vi "GetLibVersionInfo.vi"(8 "error in (no error)":errorcluster, 11 "DLLPath":path) -> (0 "error out":errorcluster, 3 "LibInfo":T1)   [LabVIEW 2022 SP3, in "EClib functions.lvlib"]
doc: "This VI supplies information on the selected DLL:\n- DLL version\n- DLL version string length\n- DLL path"
uses:
  EClib functions.lvlib
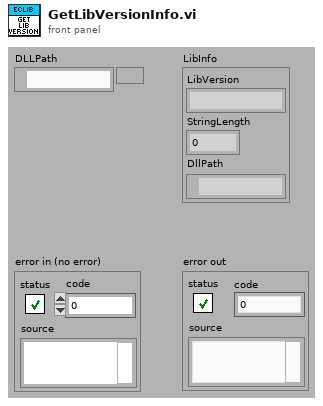
[diagram p1: front panel]
types:
  T1 = cluster{"LibVersion":string, "StringLength":u32, "DllPath":path}
  T2 = cluster{"arg1":string, "arg2":u32, "ECLibDLLPath":path}
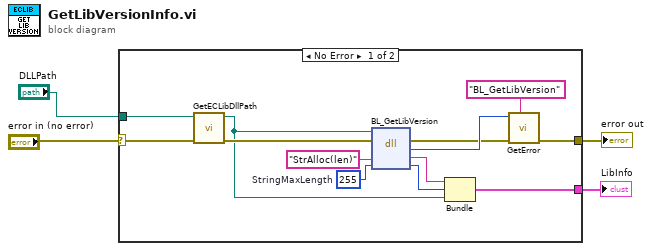
[diagram p0: block diagram]
diagram:
  n1 = case shown="No Error" "error in (no error)" {
    selector: "error in (no error)" -> [w13 w18]
    tunnel: [w17 w18] -> w3
    tunnel: [w8 _] -> w2
    tunnel: "DLLPath" -> [w5 _]
    frame No Error {
      w11 = u32 255  # StringMaxLength
      n2 = call "GetECLibDllPath.vi"("error in (no error)"=w13, "DLLPath"=w5) -> ("error out"=w12:errorcluster, "ECLibDLLPath"=w6:path)  [unwired: 8 in]
      n3 = dll-call lib="?" fn="BL_GetLibVersion"(path in=w6, error in=w12, "arg1"="StrAlloc(len)", "arg2"=w11) -> (error out=w15:errorcluster, "return type"=w16:i32, "arg1"=w10:string, "arg2"=w9:u32)  [unwired: 1 in, 1 out]
      n4 = Bundle("arg1"=w10, "arg2"=w9, "ECLibDLLPath"=w6) -> (w8:T2)  [unwired: 1 in]
      n5 = call "GetError.vi"("DLLFunction"="BL_GetLibVersion", "error in"=w15, "code"=w16) -> ("error out"=w17:errorcluster)  [unwired: 8 in]
    }
    frame Error {
    }
  }
  "error out" <- w3
  "LibInfo" <- w2
